vi "MQTT_Read_Subscribed_Topics.vi"(8 "error in (no error)":errorcluster) -> (0 "error out":errorcluster)   [LabVIEW 2025, in "DAQIO MQTT.lvlib"]
doc: "A basic example that reads topics that the client subcribed to. \n\n© 2015 - daq.io, LLC - Peter Adelhardt"
uses:
  DAQIO MQTT.lvlib
  Controls/Connection_Return_Codes.ctl
  Controls/Connect_Flags.ctl
  Controls/QoS.ctl
  Controls/DUP_Flag.ctl
  Controls/Retain_Flag.ctl
  Controls/User_Info.ctl
panel:
  out "Connection Status":T1=enum."Connection refused: not authorized"
  in  "Exit":bool
  in  "MQTT Broker":cluster{"address (IP)":string, "port":u16}={"address (IP)"="broker.hivemq.com", "port"=1883}
  out "Message IDs":u16[](array[numeric]) format="%x"
  out "Topics":string[](array[string])
  out "Messages":string[](array[string])
  in  "Client ID":string="LVSubscribeClient"
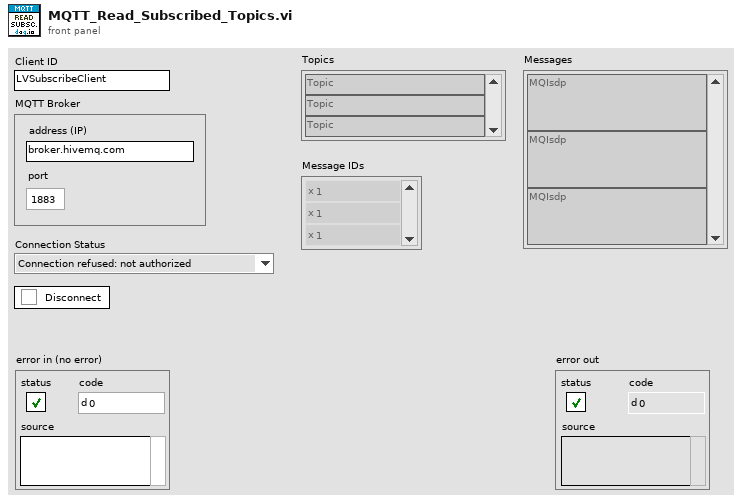
[diagram p1: front panel]
types:
  T1 = typedef "DAQIO MQTT.lvlib/Connection_Return_Codes.ctl" = enum16{"Connection accepted", "Connection refused: unacceptable protocol version", "Connection refused: identifier rejected", "Connection refused: Server unavailable", "Connection refused: bad user name or password", "Connection refused: not authorized"}
  T2 = typedef "DAQIO MQTT.lvlib/User_Info.ctl" = cluster{"User Name":string, "Password":string}
  T3 = typedef "DAQIO MQTT.lvlib/QoS.ctl" = enum8{"At most once", "At least once", "Exactly once", "Reserved"}
  T4 = typedef "DAQIO MQTT.lvlib/DUP_Flag.ctl" = bool
  T5 = typedef "DAQIO MQTT.lvlib/Retain_Flag.ctl" = bool
  T6 = cluster{"QoS":T3, "DUP":T4, "Retain":T5, "Keep Alive (sec)":u16}
  T7 = typedef "DAQIO MQTT.lvlib/Connect_Flags.ctl" = cluster{"user name":bool, "password":bool, "will retain":bool, "will flag":bool, "clean session":bool, "reserved":bool, "will QoS":T3}
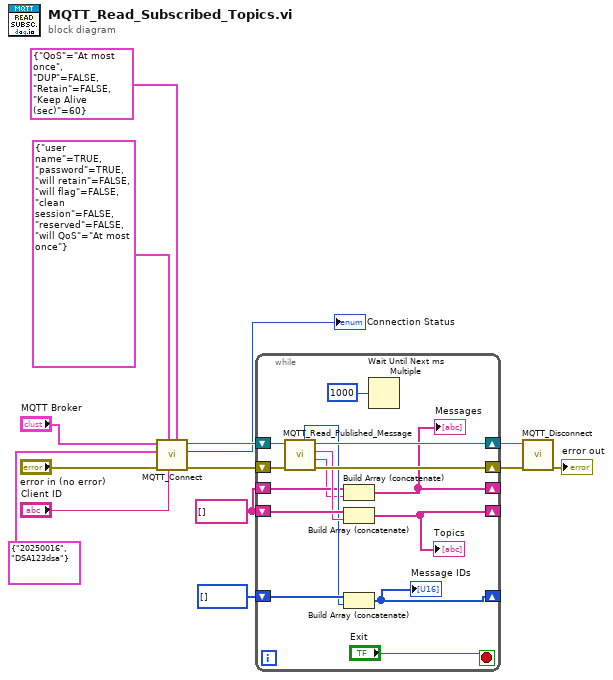
[diagram p0: block diagram]
diagram:
  w7 = string[] []
  n1 = call "MQTT_Connect.vi"("Connect Meta"=T6 {"QoS"=enum."At most once", "DUP"=FALSE, "Retain"=FALSE, "Keep Alive (sec)"=60}, "Client ID"="Client ID", "Connect Flags"=T7 {"user name"=TRUE, "password"=TRUE, "will retain"=FALSE, "will flag"=FALSE, "clean session"=FALSE, "reserved"=FALSE, "will QoS"=enum."At most once"}, "error in (no error)"="error in (no error)", "User Info"=T2 {"User Name"="20250016", "Password"="DSA123dsa"}, "MQTT Broker"="MQTT Broker") -> ("error out"=w2:errorcluster, "Connection Status"=→"Connection Status":T1, "connection ID out"=w4:refnum<k5>)  [unwired: 3 in]
  n2 = while {
    shift-right: [w24] -> w9
    shift-left: w2 -> [w26]
    shift-right: [w15] -> _
    shift-left: u16[] [] -> [w21]
    shift-right: [w16] -> _
    shift-left: w7 -> [w19]
    shift-right: [w17] -> _
    shift-left: w7 -> [w23]
    shift-right: [w25] -> w10
    shift-left: w4 -> [w27]
    stop <- "Exit" stop-if-true
    n3 = call "MQTT_Read_Published_Message.vi"("error in (no error)"=w26, "connection ID"=w27) -> ("error out"=w24:errorcluster, "Message"=w18:string, "Topic Name"=w22:string, "connection ID out"=w25:refnum<k5>, "Message ID"=w20:u16)  [unwired: 4 in, 1 out]
    n4 = Build Array (concatenate)(w19, w18) -> (w16:string[])
    "Messages" <- w16
    n5 = Build Array (concatenate)(w23, w22) -> (w17:string[])
    "Topics" <- w17
    n6 = Build Array (concatenate)(w21, w20) -> (w15:u16[])
    "Message IDs" <- w15
    n7 = Wait Until Next ms Multiple(millisecond multiple=u32 1000) -> ()  [unwired: 1 out]
  }
  n8 = call "MQTT_Disconnect.vi"("error in (no error)"=w9, "connection ID"=w10) -> ("error out"=→"error out":errorcluster)  [unwired: 9 in]
